vi "StripHeading.vi"(7 "Header":string, 9 "Padding":string, 11 "Resource in":string) -> (3 "Resource out":string)   [LabVIEW 2020]
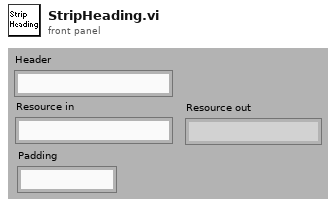
[diagram p1: front panel]
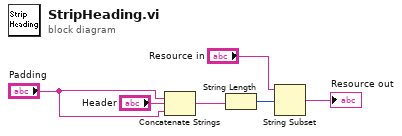
[diagram p0: block diagram]
diagram:
  n1 = Concatenate Strings("Padding", "Header", "Padding") -> (w2:string)
  n2 = String Length(string=w2) -> (length=w4:i32)
  n3 = String Subset(string="Resource in", offset (0)=w4) -> (substring=→"Resource out":string)  [unwired: 1 out]
